vi "UTILITY System Time.vi"() -> (2 "Date & Time":string[][](array[string]), 3 "System Time":string[](array[string]))   [LabVIEW 2020]
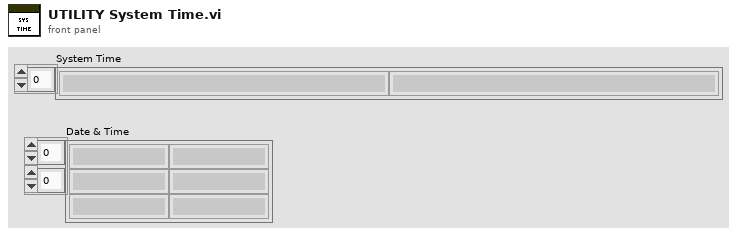
[diagram p1: front panel]
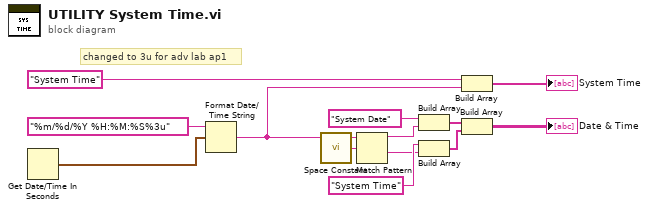
[diagram p0: block diagram]
diagram:
  # "changed to 3u for adv lab ap1"
  n1 = Get Date/Time In Seconds() -> (seconds since 1Jan1904=w11:timestamp)
  n2 = Format Date/Time String(time format string (%c)="%m/%d/%Y %H:%M:%S%3u", seconds (now)=w11) -> (date/time string=w9:string)  [unwired: 1 in]
  n3 = call <vilib>:"Space Constant.vi"() -> ("String"=w10:string)
  n4 = Match Pattern(string=w9, regular expression=w10) -> (before substring=w8:string, after substring=w5:string)  [unwired: 1 in, 2 out]
  n5 = Build Array("System Date" ("element"), w8) -> (w4:string[])
  n6 = Build Array("System Time" ("element"), w5) -> (w3:string[])
  n7 = Build Array("System Time" ("element"), w9) -> (→"System Time":string[])
  n8 = Build Array(w4, w3) -> (→"Date & Time":string[][])
